vi "Msg EnQ.vi"(6 "Priority?":bool, 9 "Msg":refnum<class "Msg.lvclass">, 10 "Msg Q":refnum<queue>) -> (0 "error out":errorcluster)   [LabVIEW 2021, in "LVCAM.lvlib" / "Self Actor.lvclass"]
uses:
  Self Actor.lvclass
  Msg/Msg.lvclass
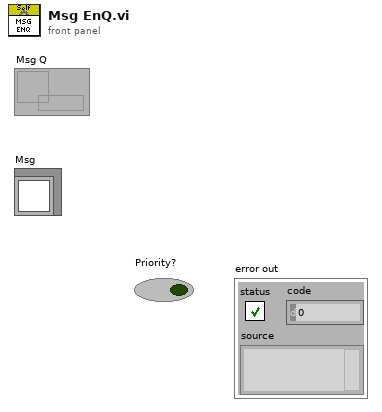
[diagram p1: front panel]
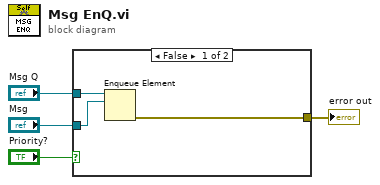
[diagram p0: block diagram]
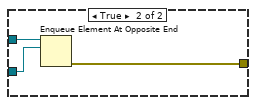
[diagram p2: hidden frame]
diagram:
  n1 = case shown="False" "Priority?" {
    tunnel: [w7 w8] -> w3
    tunnel: "Msg Q" -> [w6 w10]
    tunnel: "Msg" -> [w5 w9]
    frame False {
      n2 = Enqueue Element(queue=w6, element=w5) -> (error out=w7:errorcluster)  [unwired: 2 in, 2 out]
    }
    frame True {
      n3 = Enqueue Element At Opposite End(queue=w10, element=w9) -> (error out=w8:errorcluster)  [unwired: 2 in, 2 out]
    }
  }
  "error out" <- w3
